vi "DraftOCU2.vi"() -> ()   [LabVIEW 2013]
uses:
  cRIO_Code/Data/TypeDefs/MissionTypeControl.ctl
  cRIO_Code/Data/TypeDefs/UTM Location.ctl
  cRIO_Code/Data/TypeDefs/MissionDescription.ctl
  cRIO_Code/Logic/Classes/Missions/GenericMission/GenericMission.lvclass
  Location of Think.ctl
  RIO-OCU_Comm/ToRIO.ctl
  CommandMessages.ctl
  cRIO_Code/Logic/Classes/Missions/GoTo/GoTo.lvclass
  cRIO_Code/Logic/Classes/Missions/RoundBouy/RoundBouy.lvclass
  cRIO_Code/Logic/Classes/Missions/PassBouy/PassBouy.lvclass
  cRIO_Code/Logic/Classes/Missions/StationKeeping/StationKeeping.lvclass
  RIO-OCU_Comm/NetworkStreams/Writer/NetworkStreamWriter.lvclass
panel:
  in  "DeleteMission":bool
  out "Current Missions":T1[](array[typedef]) {"Points of Interest"."North" format="%#_10f"; "Points of Interest"."East" format="%#_8f"}
  out "# of Missions":i32
  in  "ID# To Delete":u16
  in  "stop":bool
  in  "Timeout (s)":dbl=-1.0
  in  "Duration (s)":dbl=-1.0
  in  "Tolerance (m)":dbl
  in  "Points of Interest":T3[](array[typedef]) {"North" format="%#_10f"; "East" format="%#_8f"}
  in  "Mission Type":T2
  in  "CreateMission":bool
  # "TODO: Add in the clickable map"
  # "TODO: When you delete the last mission, make idle take its place. Then when the next mission is initialized, delete the idle mission"
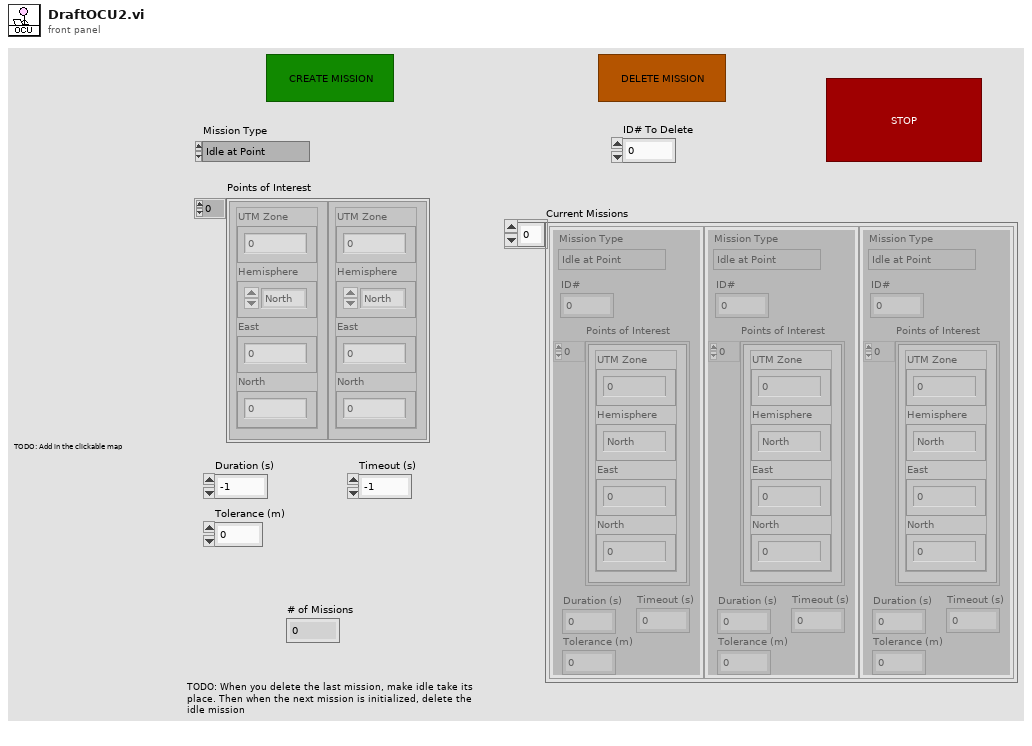
[diagram p1: front panel]
types:
  T1 = typedef "MissionDescription.ctl" = cluster{"Duration (s)":dbl, "Timeout (s)":dbl, "Tolerance (m)":dbl, "Mission Type":T2, "Points of Interest":T3[], "ID#":i32}
  T2 = typedef "MissionTypeControl.ctl" = enum16{"Idle at Point", "Drive to Waypoint", "Round Buoy to Port", "Round Buoy to Starboard", "Pass Between Buoys", "Station Keeping"}
  T3 = typedef "UTM Location.ctl" = cluster{"UTM Zone":dbl, "Hemisphere":enum16{"North", "South"}, "East":dbl, "North":dbl}
  T4 = typedef "Location of Think.ctl" = string
  T5 = typedef "CommandMessages.ctl" = enum16{"OverrideMode", "Add mission", "Delete mission", "Change constants"}
  T6 = typedef "ToRIO.ctl" = cluster{"String":string, "Commands":T5}
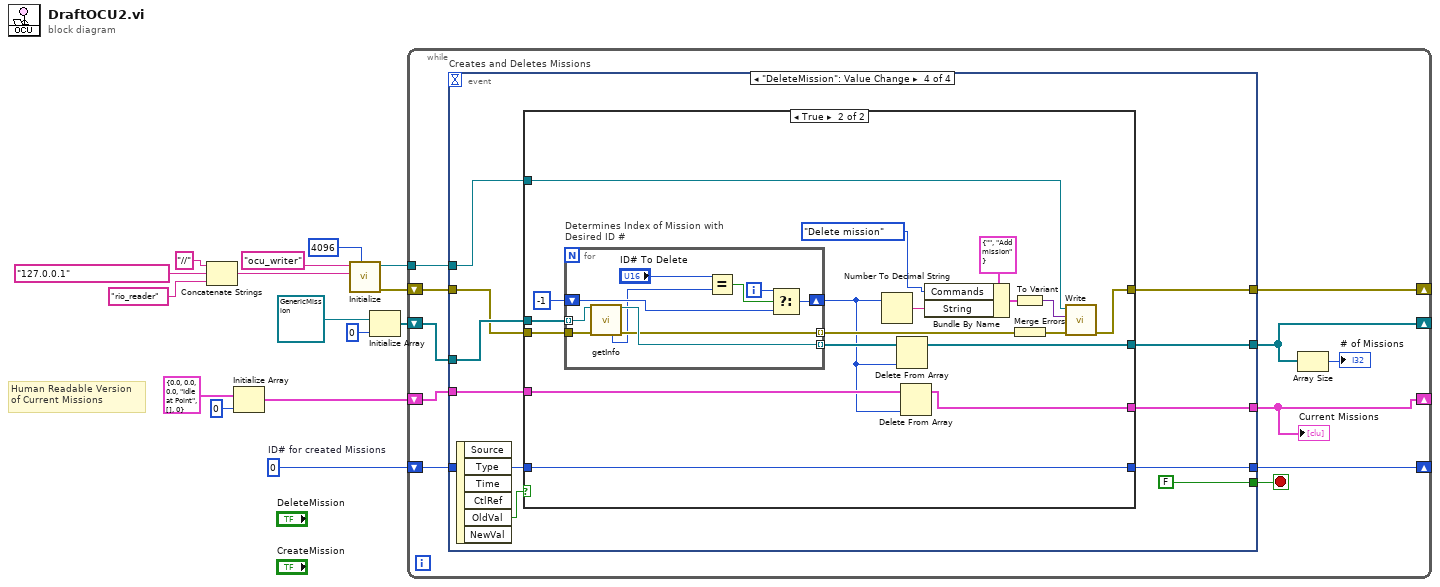
[diagram p0: block diagram]
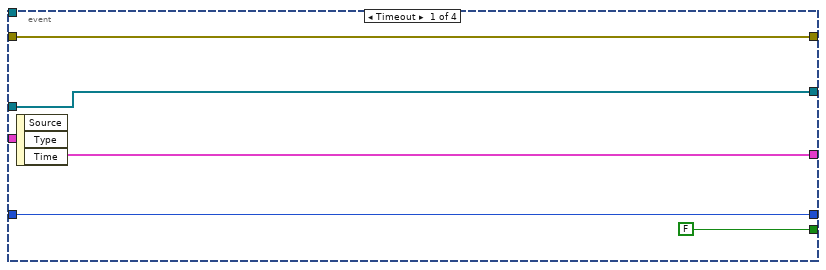
[diagram p2: hidden frame]
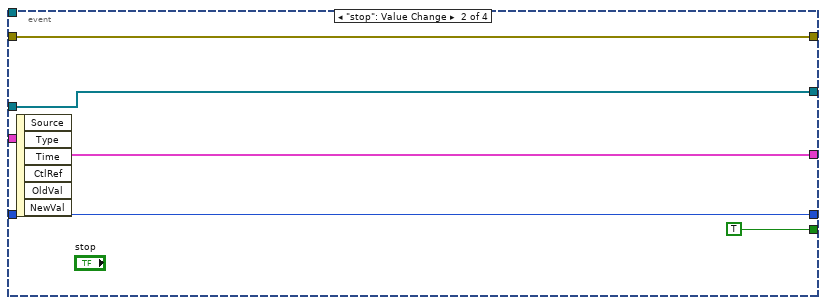
[diagram p3: hidden frame]
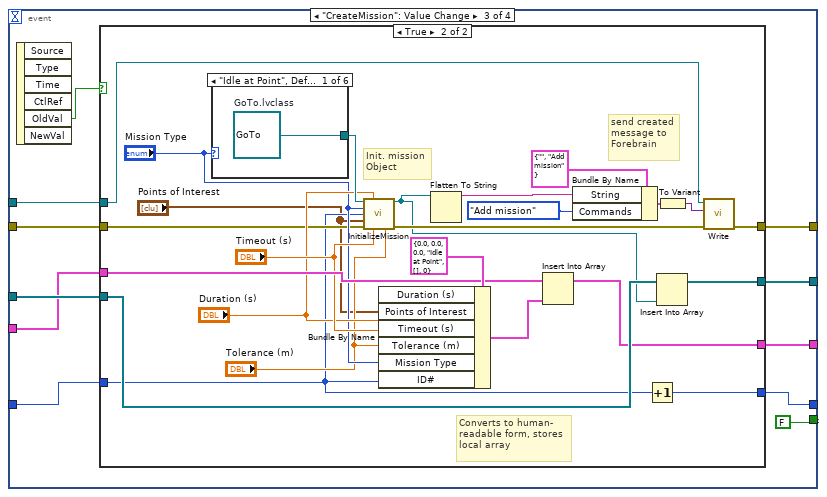
[diagram p4: hidden frame]
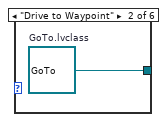
[diagram p6: hidden frame]
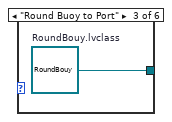
[diagram p7: hidden frame]
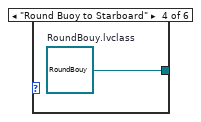
[diagram p8: hidden frame]
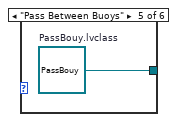
[diagram p9: hidden frame]
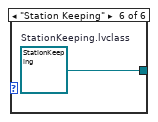
[diagram p10: hidden frame]
diagram:
  w13 = 0  # ID# for created Missions
  # "Human Readable Version\nof Current Missions"
  n1 = Concatenate Strings("//" ("string"), T4 "127.0.0.1" ("Location of THINK"), "rio_reader" ("string")) -> (w3:string)
  n2 = Initialize Array(T1 {"Duration (s)"=0.0, "Timeout (s)"=0.0, "Tolerance (m)"=0.0, "Mission Type"=enum."Idle at Point", "Points of Interest"=[], "ID#"=0} ("input cluster"), 0 ("dimension size")) -> (w10:T1[])
  n3 = call "Initialize.vi"("writer buffer size"=4096, "reader url"=w3, "writer name"="ocu_writer") -> ("error out"=w1:errorcluster, "NetworkStreamWriter out"=w2:refnum<class "NetworkStreamWriter.lvclass">)  [unwired: 7 in]
  n4 = Initialize Array(refnum<class "GenericMission.lvclass"> refnum ("GenericMission.lvclass"), 0 ("dimension size")) -> (w14:refnum<class "GenericMission.lvclass">[])
  n5 = while {
    shift-right: [w20] -> _
    shift-left: w14 -> [w26]
    shift-right: [w24] -> _
    shift-left: w13 -> [w25]
    shift-right: [w21] -> _
    shift-left: w10 -> [w22]
    tunnel: w2 -> [w17]
    shift-right: [w18] -> _
    shift-left: w1 -> [w16]
    stop <- w19 stop-if-true
    n6 = event "Creates and Deletes Missions" shown="[3] \"DeleteMission\": Value Change" {
      selector: _ -> [_ _ _ _]
      dyn-events: _ -> [_ _ _ _]
      timeout: _ -> [_ _ _ _]
      tunnel: w26 -> [w30 w35 w46 w92]
      tunnel: [w30 w35 w45 w91] -> w20
      tunnel: w25 -> [w31 w34 w47 w86]
      tunnel: [w31 w34 w41 w87] -> w24
      tunnel: w22 -> [w28 w33 w44 w90]
      tunnel: [w28 w33 w43 w89] -> w21
      tunnel: [FALSE TRUE FALSE FALSE] -> w19
      tunnel: [w27 w32 w39 w84] -> w18
      tunnel: w17 -> [_ _ w38 w82]
      tunnel: w16 -> [w27 w32 w37 w83]
      event Timeout {
        n7 = event-data() -> ()  [unwired: 1 in, 3 out]
      }
      event "stop": Value Change {
        n8 = event-data() -> ()  [unwired: 1 in, 6 out]
      }
      event "CreateMission": Value Change {
        n9 = event-data() -> ("OldVal"=w40:bool)  [unwired: 1 in, 5 out]
        n10 = case shown="True" w40 {
          tunnel: w47 -> [w49 w53]
          tunnel: w46 -> [w51 w74]
          tunnel: [w51 w73] -> w45
          tunnel: w44 -> [w50 w70]
          tunnel: [w50 w69] -> w43
          tunnel: [w49 w64] -> w41
          tunnel: [w48 w63] -> w39
          tunnel: w38 -> [_ w61]
          tunnel: w37 -> [w48 w60]
          frame False {
          }
          frame True {
            # "Init. mission\nObject"
            # "send created\nmessage to\nForebrain"
            # "Converts to human-\nreadable form, stores\nlocal array"
            n11 = case shown="\"Idle at Point\", Default" "Mission Type" {
              tunnel: [w76 w77 w78 w79 w80 w81] -> w75
              frame "Idle at Point", Default {
                w76 = refnum<class "GoTo.lvclass"> refnum  # GoTo.lvclass
              }
              frame "Drive to Waypoint" {
                w77 = refnum<class "GoTo.lvclass"> refnum  # GoTo.lvclass
              }
              frame "Round Buoy to Port" {
                w78 = refnum<class "RoundBouy.lvclass"> refnum  # RoundBouy.lvclass
              }
              frame "Round Buoy to Starboard" {
                w79 = refnum<class "RoundBouy.lvclass"> refnum  # RoundBouy.lvclass
              }
              frame "Pass Between Buoys" {
                w80 = refnum<class "PassBouy.lvclass"> refnum  # PassBouy.lvclass
              }
              frame "Station Keeping" {
                w81 = refnum<class "StationKeeping.lvclass"> refnum  # StationKeeping.lvclass
              }
            }
            n12 = call-dynamic "InitializeMission.vi"("GenericMission in"=w75, "Duration (s)"="Duration (s)", "Mission Type"="Mission Type", "ID#"=w53, "Points of Interest"="Points of Interest", "Error In"=w60, "Timeout (s)"="Timeout (s)", "Tolerance (m)"="Tolerance (m)") -> ("GenericMission out"=w57:refnum<class "GenericMission.lvclass">, "Error Out"=w62:errorcluster)  [unwired: 6 in]
            n13 = Bundle By Name(cluster=T1 {"Duration (s)"=0.0, "Timeout (s)"=0.0, "Tolerance (m)"=0.0, "Mission Type"=enum."Idle at Point", "Points of Interest"=[], "ID#"=0} ("input cluster"), "Duration (s)"="Duration (s)", "Points of Interest"="Points of Interest", "Timeout (s)"="Timeout (s)", "Tolerance (m)"="Tolerance (m)", "Mission Type"="Mission Type", "ID#"=w53) -> (w71:T1)
            n14 = Flatten To String(anything=w57) -> (data string=w59:string)  [unwired: 3 in, 2 out]
            n15 = Insert Into Array(array=w70, new element=w71) -> (w69:T1[])  [unwired: 1 in]
            n16 = Bundle By Name(cluster=T6 {"String"="", "Commands"=enum."Add mission"} ("To RIO"), "String"=w59, "Commands"=CommandMessages."Add mission") -> (w54:T6)
            n17 = Increment(x=w53) -> (x+1=w64:i32)
            n18 = Insert Into Array(array=w74, new element=w57) -> (w73:refnum<class "GenericMission.lvclass">[])  [unwired: 1 in]
            n19 = To Variant(anything=w54) -> (Variant=w55:variant)
            n20 = call "Write.vi"("error in (no error)"=w62, "element"=w55, "NetworkStreamWriter in"=w61) -> ("error out"=w63:errorcluster)  [unwired: 7 in, 1 out]
          }
        }
      }
      event "DeleteMission": Value Change {
        n21 = event-data() -> ("OldVal"=w85:bool)  [unwired: 1 in, 5 out]
        n22 = case shown="True" w85 {
          tunnel: w92 -> [w96 w114]
          tunnel: [w96 w111] -> w91
          tunnel: w90 -> [w95 w110]
          tunnel: [w95 w109] -> w89
          tunnel: [w94 w108] -> w87
          tunnel: w86 -> [w94 w108]
          tunnel: [w93 w99] -> w84
          tunnel: w83 -> [w93 w98]
          tunnel: w82 -> [_ w97]
          frame False {
          }
          frame True {
            n23 = for "Determines Index of Mission with\nDesired ID #" {
              tunnel: w114 -> [w124] mode=indexing
              tunnel: [w123] -> w112 mode=indexing
              shift-right: [w120] -> w106
              shift-left: -1 -> [w119]
              tunnel: [w118] -> w107 mode=indexing
              tunnel: w98 -> [w117]
              i -> [w121]
              n24 = call-dynamic "getInfo.vi"("GenericMission in"=w124, "error in (no error)"=w117) -> ("GenericMission out"=w123:refnum<class "GenericMission.lvclass">, "ID#"=w115:u16, "error out"=w118:errorcluster)  [unwired: 5 in, 6 out]
              n25 = Equal?(x="ID# To Delete", y=w115) -> (x = y?=w122:bool)
              n26 = Select(t=w121, s=w122, f=w119) -> (s? t:f=w120:i32)
            }
            n27 = Number To Decimal String(number=w106) -> (decimal integer string=w101:string)  [unwired: 1 in]
            n28 = Delete From Array(array=w112, index=w106) -> (array with subset deleted=w111:refnum<class "GenericMission.lvclass">[])  [unwired: 1 in, 1 out]
            n29 = Delete From Array(array=w110, index=w106) -> (array with subset deleted=w109:T1[])  [unwired: 1 in, 1 out]
            n30 = Bundle By Name(cluster=T6 {"String"="", "Commands"=enum."Add mission"} ("To RIO"), "Commands"=CommandMessages."Delete mission", "String"=w101) -> (w104:T6)
            n31 = To Variant(anything=w104) -> (Variant=w103:variant)
            n32 = Merge Errors(w107) -> (w102:errorcluster)
            n33 = call "Write.vi"("error in (no error)"=w102, "element"=w103, "NetworkStreamWriter in"=w97) -> ("error out"=w99:errorcluster)  [unwired: 7 in, 1 out]
          }
        }
      }
    }
    "Current Missions" <- w21
    n34 = Array Size(array=w20) -> (size(s)=→"# of Missions":i32)
  }
